vi "temp_VI_UnderTest.vi"(8 "error in":errorcluster) -> (0 "error out":errorcluster, 2 "actual result":string)   [LabVIEW 2019, in "TestVoting.lvclass"]
uses:
  TestVoting.lvclass
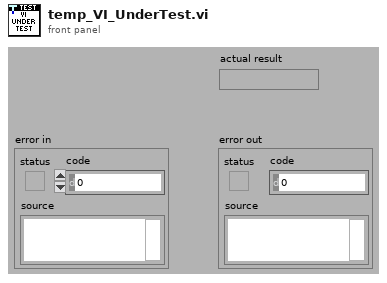
[diagram p1: front panel]
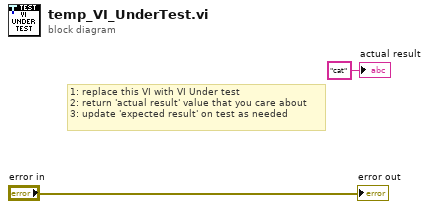
[diagram p0: block diagram]
diagram:
  # "1: replace this VI with VI Under test\n2: return 'actual result' value that you care about\n3: update 'expected result' on test as needed"
  "error out" <- "error in"
  "actual result" <- "cat" ("actual result")
